vi "initialize python session.vi"(8 "error in (no error)":errorcluster, 11 "Save Image in":refnum<class "Save Image.lvclass">) -> (0 "error out":errorcluster, 3 "Save Image out":refnum<class "Save Image.lvclass">)   [LabVIEW 2018, in "Save Image.lvclass"]
doc: "Initialize the Python Toolkit"
uses:
  Save Image.lvclass
  Save Image.lvclass/Save Image.ctl
  Python Toolkit/Python Toolkit.lvclass
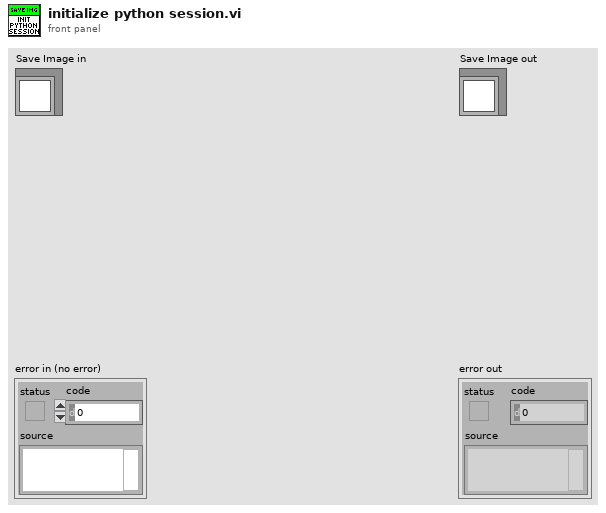
[diagram p1: front panel]
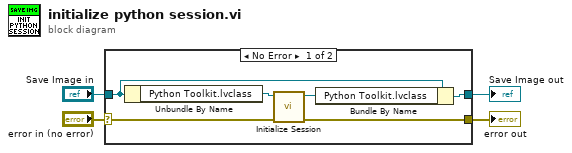
[diagram p0: block diagram]
diagram:
  n1 = case shown="No Error" "error in (no error)" {
    selector: "error in (no error)" -> [w7 w12]
    tunnel: [w5 w12] -> w3
    tunnel: [w9 w11] -> w1
    tunnel: "Save Image in" -> [w8 w11]
    frame No Error {
      n2 = Unbundle By Name(w8) -> ("Python Toolkit.lvclass"=w10:refnum<class "Python Toolkit.lvclass">)
      n3 = call "Initialize Session.vi"("error in (no error)"=w7, "Python Toolkit in"=w10) -> ("error out"=w5:errorcluster, "Python Toolkit out"=w6:refnum<class "Python Toolkit.lvclass">)  [unwired: 8 in]
      n4 = Bundle By Name(cluster=w8, "Python Toolkit.lvclass"=w6) -> (w9:refnum<class "Save Image.lvclass">)
    }
    frame Error {
    }
  }
  "error out" <- w3
  "Save Image out" <- w1
